vi "readbin(dbl).vi"(9 "Legnth":i32=8, 10 "Offset":i32, 11 "Buffer INÂ":string) -> (1 "Double":dbl format="%.3f", 2 "Offset+Length":i32, 3 "Buffer OUT":string)   [LabVIEW 2017, in "HEKAdat.lvclass"]
uses:
  HEKAdat.lvclass
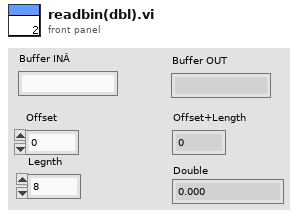
[diagram p1: front panel]
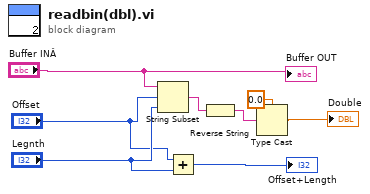
[diagram p0: block diagram]
diagram:
  n1 = String Subset(string="Buffer INÂ", offset (0)="Offset", length (rest)="Legnth") -> (substring=w1:string)
  n2 = Add(x="Offset", y="Legnth") -> (x+y=→"Offset+Length":i32)
  n3 = Reverse String(1:w1) -> (0:w3:string)
  n4 = Type Cast(type=0.0 ("오프셋(0)"), x=w3) -> (*(type *) &x=→"Double":dbl)
  "Buffer OUT" <- "Buffer INÂ"
